vi "CLOCK.vi"() -> ()   [LabVIEW 2018]
panel:
  in  "停止按钮":bool
  out "Minute":i32(knob) scale=0.0..60.0
  out "Second":i32(knob) scale=0.0..60.0
  out "Hour":i32(knob) scale=0.0..720.0
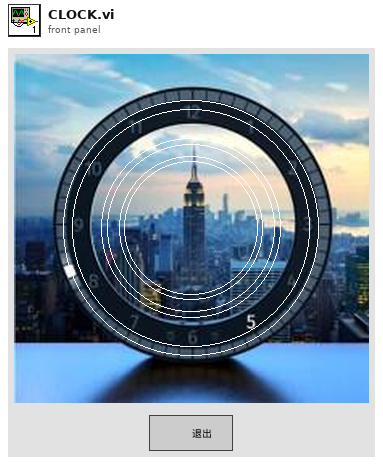
[diagram p1: front panel]
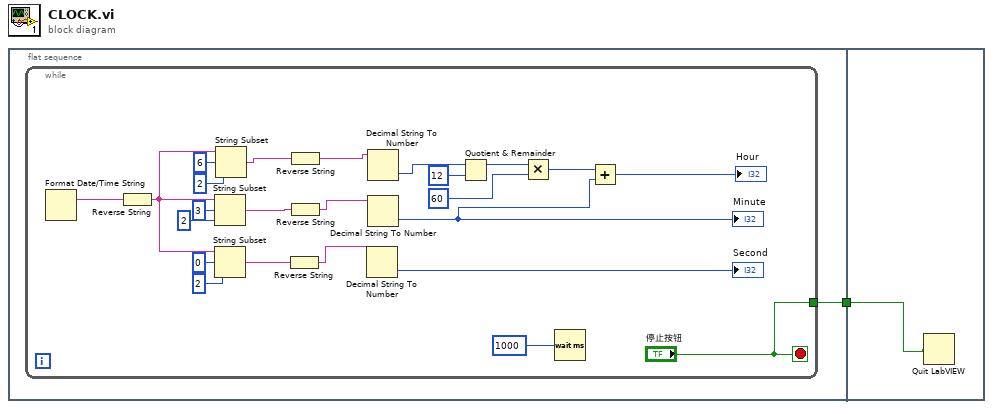
[diagram p0: block diagram]
diagram:
  n1 = flat-sequence {
    tunnel: [w2] -> w1
    tunnel: w1 -> [w27]
    frame #0 {
      n2 = while {
        tunnel: ["停止按钮"] -> w2
        stop <- "停止按钮" stop-if-true
        n3 = Format Date/Time String() -> (date/time string=w13:string)  [unwired: 3 in]
        n4 = Reverse String(1:w13) -> (0:w26:string)
        n5 = String Subset(string=w26, offset (0)=3 ("偏移量(0)"), length (rest)=2 ("长度（剩余）")) -> (substring=w17:string)
        n6 = String Subset(string=w26, offset (0)=0 ("偏移量(0)"), length (rest)=2 ("长度（剩余）")) -> (substring=w15:string)
        n7 = String Subset(string=w26, offset (0)=6 ("偏移量(0)"), length (rest)=2 ("长度（剩余）")) -> (substring=w19:string)
        n8 = Reverse String(1:w15) -> (0:w14:string)
        n9 = Reverse String(1:w19) -> (0:w18:string)
        n10 = Reverse String(1:w17) -> (0:w16:string)
        n11 = Decimal String To Number(string=w14) -> (number=→"Second":i32)  [unwired: 2 in, 1 out]
        n12 = Decimal String To Number(string=w18) -> (number=w22:i32)  [unwired: 2 in, 1 out]
        n13 = Decimal String To Number(string=w16) -> (number=w3:i32)  [unwired: 2 in, 1 out]
        "Minute" <- w3
        n14 = Quotient & Remainder(x=w22, y=12) -> (x-y*floor(x/y)=w7:i32)  [unwired: 1 out]
        n15 = Multiply(x=w7, y=60) -> (x*y=w5:i32)
        n16 = Wait (ms)(milliseconds to wait=u32 1000 ("毫秒计时值")) -> ()  [unwired: 1 out]
        n17 = Add(x=w5, y=w3) -> (x+y=→"Hour":i32)
      }
    }
    frame #1 {
      n18 = Quit LabVIEW(quit? (T)=w27) -> ()
    }
  }
